vi "FG Queue.vi"(2 "FG Action":enum16{"Read", "Write"}(ring), 3 "queue in":refnum<queue>) -> (1 "queue out":refnum<queue>)   [LabVIEW 2009]
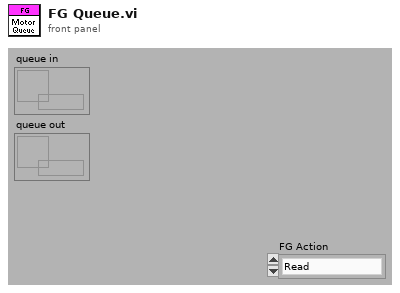
[diagram p1: front panel]
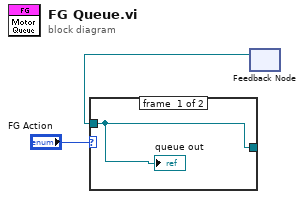
[diagram p0: block diagram]
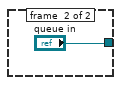
[diagram p2: hidden frame]
diagram:
  n1 = feedback #1() -> (w1:refnum<queue>)  [unwired: 1 in]
  n2 = case shown="\"Read\", Default" "FG Action" {
    tunnel: [w4 "queue in"] -> w2
    tunnel: w1 -> [w4 _]
    frame #0 {
      "queue out" <- w4
    }
    frame #1 {
    }
  }
